vi "example (feedback node).vi"() -> ()   [LabVIEW 2021]
panel:
  out "Tank":dbl(slide) scale=0.0..10.0
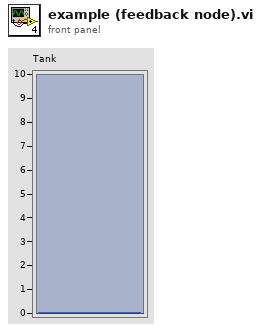
[diagram p1: front panel]
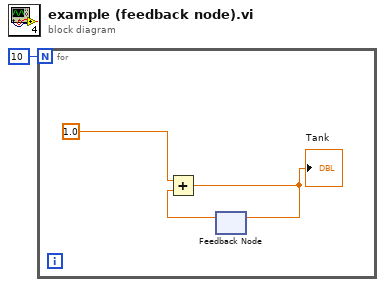
[diagram p0: block diagram]
diagram:
  n1 = for {
    N: 10 -> [_]
    n2 = feedback #1() -> (w3:dbl)  [unwired: 1 in]
    n3 = Add(x=1.0, y=w3) -> (x+y=w2:dbl)
    "Tank" <- w2
    n4 = feedback-in #1(w2) -> ()
  }
